vi "Start Execution Event Callback.vi"(4 "TS UI Data":T1, 5 "Event Data":T2, 6 "Control Ref":refnum<k7>, 7 "Event Common Data":T3) -> ()   [LabVIEW 2015]
uses:
  Type defs/TS UI Data.ctl
  Type defs/Nest cluster.ctl
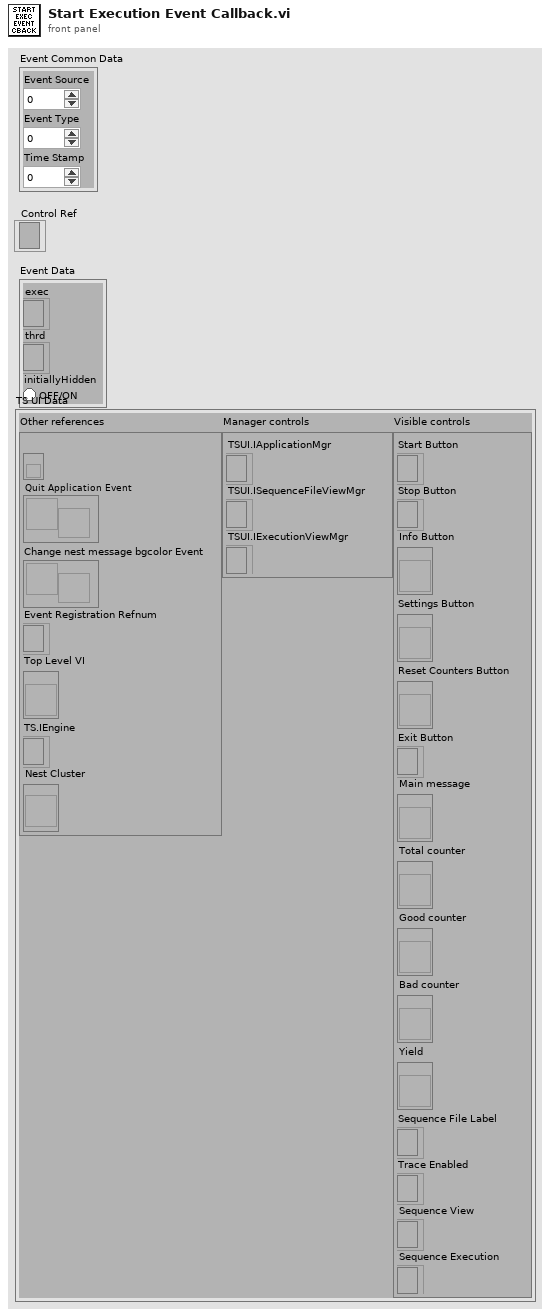
[diagram p1: front panel]
types:
  T1 = typedef "TS UI Data.ctl" = cluster{"Other references":cluster{"event callback refnum":refnum<k27>, "Quit Application Event":refnum<user-event>, "Change nest message bgcolor Event":refnum<user-event>, "event registration refnum":refnum<event-registration>, "Top Level VI":refnum<vi>, "TS.IEngine":refnum<k7>, "Nest Cluster":refnum<vi>}, "Manager controls":cluster{"TSUI.IApplicationMgr":refnum<k7>, "TSUI.ISequenceFileViewMgr":refnum<k7>, "TSUI.IExecutionViewMgr":refnum<k7>}, "Visible controls":cluster{"Start Button":refnum<k7>, "Stop Button":refnum<k7>, "Info Button":refnum<vi>, "Settings Button":refnum<vi>, "Reset Counters Button":refnum<vi>, "Exit Button":refnum<k7>, "Main message":refnum<vi>, "Total counter":refnum<vi>, "Good counter":refnum<vi>, "Bad counter":refnum<vi>, "Yield":refnum<vi>, "Sequence File Label":refnum<k7>, "Trace Enabled":refnum<k7>, "Sequence View":refnum<k7>, "Sequence Execution":refnum<k7>}}
  T2 = cluster{"exec":refnum<k7>, "thrd":refnum<k7>, "initiallyHidden":bool}
  T3 = cluster{"Event Source":i32, "Event Type":u32, "Time Stamp":u32}
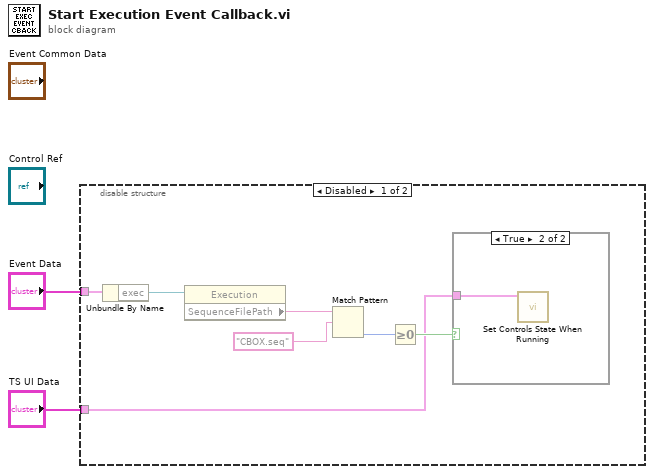
[diagram p0: block diagram]
diagram:
  n1 = disable-structure shown="Disabled" {
    disable-tunnel: "Event Data" -> [w9 _]
    disable-tunnel: "TS UI Data" -> [w3 _]
    frame Disabled {
      n2 = Unbundle By Name(w9) -> ("exec"=w8:refnum<k7>)
      n3 = property class="Execution"(reference=w8) -> ("SequenceFilePath"=w7:string)  [unwired: 1 in, 2 out]
      n4 = Match Pattern(string=w7, regular expression="CBOX.seq") -> (offset past match=w5:i32)  [unwired: 1 in, 3 out]
      n5 = Greater Or Equal To 0?(x=w5) -> (x >= 0?=w4:bool)
      n6 = case shown="True" w4 {
        tunnel: w3 -> [_ w10]
        frame False {
        }
        frame True {
          n7 = call "Set Controls State When Running.vi"("TS UI Data in"=w10) -> ()  [unwired: 10 in, 1 out]
        }
      }
    }
    frame Enabled {
    }
  }
